vi "NicmosGetDataDAQ.vi"(3 "task/channels in":refnum<k21> caption="Task In", 9 "error out":errorcluster caption="error in (no error)") -> (0 "task out":refnum<k21> caption="Task Out", 2 "NICMOS.RAW":T1, 6 "error in (no error)":errorcluster caption="error out")   [LabVIEW 2009]
uses:
  Controls/NICMOS.RAW.ctl
  <vilib>/DAQmx/read.llb/DAQmx Read (Digital 1D U16 1Chan NSamp).vi
  NicmosGlobal.vi
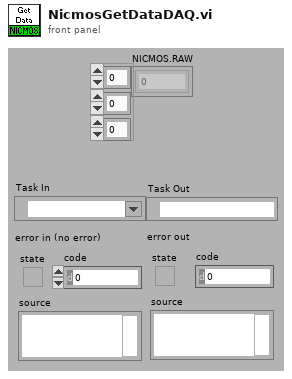
[diagram p1: front panel]
types:
  T1 = typedef "NICMOS.RAW.ctl" = u16[][][]
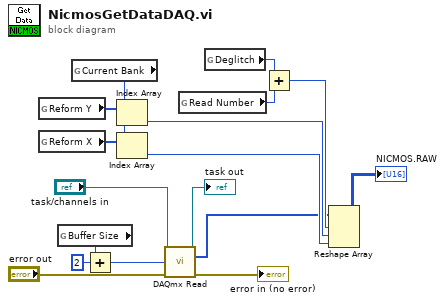
[diagram p0: block diagram]
diagram:
  n1 = global read "NicmosGlobal.vi" "Reform Y"() -> (w9:i32[])
  n2 = global read "NicmosGlobal.vi" "Reform X"() -> (w10:i32[])
  n3 = global read "NicmosGlobal.vi" "Buffer Size"() -> (w12:u32)
  n4 = global read "NicmosGlobal.vi" "Current Bank"() -> (w8:i32)
  n5 = Add(x=w12, y=2) -> (x+y=w14:u32)
  n6 = Index Array(array=w9, index=w8) -> (element=w5:i32)
  n7 = Index Array(array=w10, index=w8) -> (element=w4:i32)
  n8 = call-poly <vilib>:"DAQmx Read.vi"("task/channels in"="task/channels in", "number of samples per channel"=w14, "error in"="error out") -> ("task out"=→"task out":refnum<k21>, "data"=w2:u16[], "error out"=→"error in (no error)":errorcluster)  [unwired: 10 in]
  n9 = global read "NicmosGlobal.vi" "Read Number"() -> (w7:i32)
  n10 = global read "NicmosGlobal.vi" "Deglitch"() -> (w3:i32)
  n11 = Add(x=w3, y=w7) -> (x+y=w6:i32)
  n12 = Reshape Array(w2, w6, w5, w4) -> (→"NICMOS.RAW":u16[][][])
